vi "Equipment_Create.vi"(8 "error in (no error)":errorcluster, 9 "Cost":dbl, 10 "ID":string, 11 "reference in":refnum<class "Equipment.lvclass">) -> (0 "error out":errorcluster, 3 "reference out":refnum<class "Equipment.lvclass">)   [LabVIEW 2020, in "Equipment.lvclass"]
uses:
  Equipment.lvclass
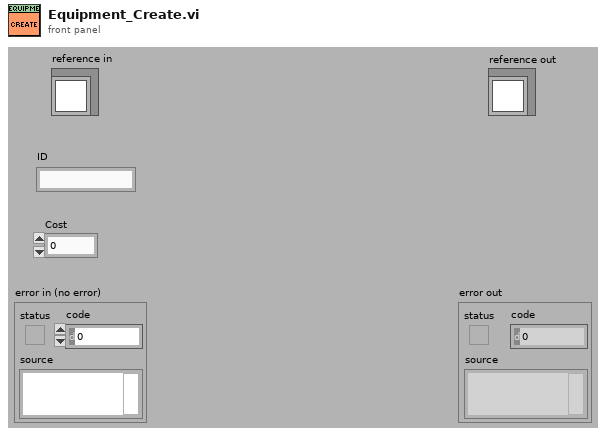
[diagram p1: front panel]
types:
  T1 = typedef "Equipment.lvclass/ObjectAttributes.ctl" = cluster{"ID":string, "Cost":dbl}
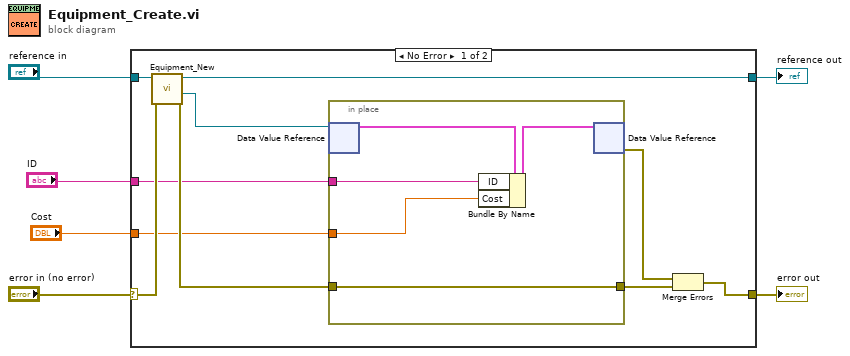
[diagram p0: block diagram]
diagram:
  n1 = case shown="No Error" "error in (no error)" {
    selector: "error in (no error)" -> [w15 w23]
    tunnel: [w12 w23] -> w5
    tunnel: "reference in" -> [w16 w22]
    tunnel: [w14 w22] -> w3
    tunnel: "ID" -> [w8 _]
    tunnel: "Cost" -> [w7 _]
    frame No Error {
      n2 = call "Equipment_New.vi"("error in (no error)"=w15, "reference in"=w16) -> ("error out"=w10:errorcluster, "DVRRefOut"=w11:refnum<data-value>, "reference out"=w14:refnum<class "Equipment.lvclass">)  [unwired: 6 in, 1 out]
      n3 = in-place {
        in-place-border: w10 -> [w19]
        in-place-border: [w19] -> w9
        in-place-border: w8 -> [w18]
        in-place-border: w7 -> [w17]
        n4 = in-place-dvr #1(w11) -> (w20:T1)  [unwired: 1 out]
        n5 = Bundle By Name(cluster=w20, "ID"=w18, "Cost"=w17) -> (w21:T1)
        n6 = in-place-dvr #1(w21) -> (w13:errorcluster)  [unwired: 1 out]
      }
      n7 = Merge Errors(w13, w9) -> (w12:errorcluster)
    }
    frame Error {
    }
  }
  "error out" <- w5
  "reference out" <- w3
